vi "PXI-Get Terminal Name with Device Prefix.vi"(8 "error in (no error)":errorcluster, 10 "Local Terminal Name":string, 11 "task/channels in":refnum<k21>) -> (0 "error out":errorcluster, 2 "Terminal Name with Device Prefix":string, 3 "task out":refnum<k21>)   [LabVIEW 2020]
doc: "This example takes in a DAQmx Task and a terminal and converts this to a terminal which includes the device prefix specified in the DAQmx Physical Channel Control.\n\nFor example: \nDAQmx Task/channels in=Dev1/ai1:2\nTerminal=ai/StartTrigger\nDevice+Terminal=/Dev1/ai/StartTrigger"
uses:
  <resource>/objmgr/daqmx.rc
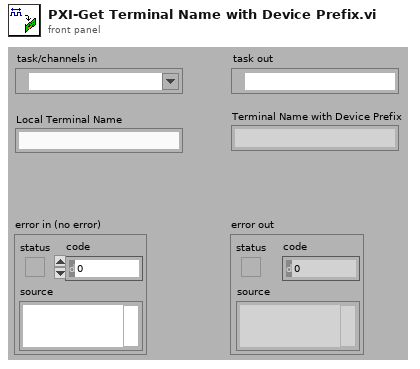
[diagram p1: front panel]
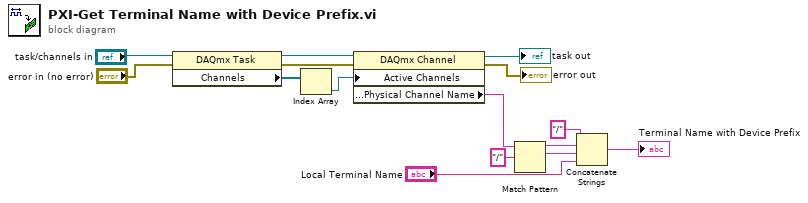
[diagram p0: block diagram]
diagram:
  n1 = property class="DAQmx Task"(reference="task/channels in", error in="error in (no error)") -> (reference out=w10:refnum<k21>, error out=w6:errorcluster, "Channels"=w9:refnum<k21>[])
  n2 = Index Array(array=w9) -> (element=w8:refnum<k21>)  [unwired: 1 in]
  n3 = property class="DAQmx Channel"(reference=w10, error in=w6, "Active Channels"=w8) -> (reference out=→"task out":refnum<k21>, error out=→"error out":errorcluster, "General Properties:Physical Channel Name"=w5:tag)
  n4 = Match Pattern(string=w5, regular expression="/") -> (before substring=w12:string, match substring=w13:string)  [unwired: 1 in, 2 out]
  n5 = Concatenate Strings("/" ("string"), w12, w13, "Local Terminal Name") -> (→"Terminal Name with Device Prefix":string)
